vi "adaptive filter NLMS(sub VI).vi"(0 "ERR":dbl=0.060310676968585164, 1 "NLMS-r(防止過大步長)":dbl=10.0, 2 "輸入訊號":dbl, 3 "order":i32=10, 5 "u(收斂係數)":dbl=0.001) -> (6 "FIR輸出":dbl=-1.0516183080382016, 7 "收斂係數u":dbl=0.060310676968585164, 8 "權重":dbl[](array[numeric]))   [LabVIEW 2010]
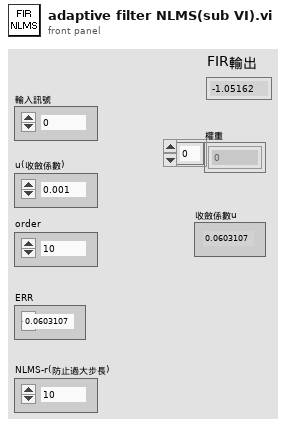
[diagram p1: front panel]
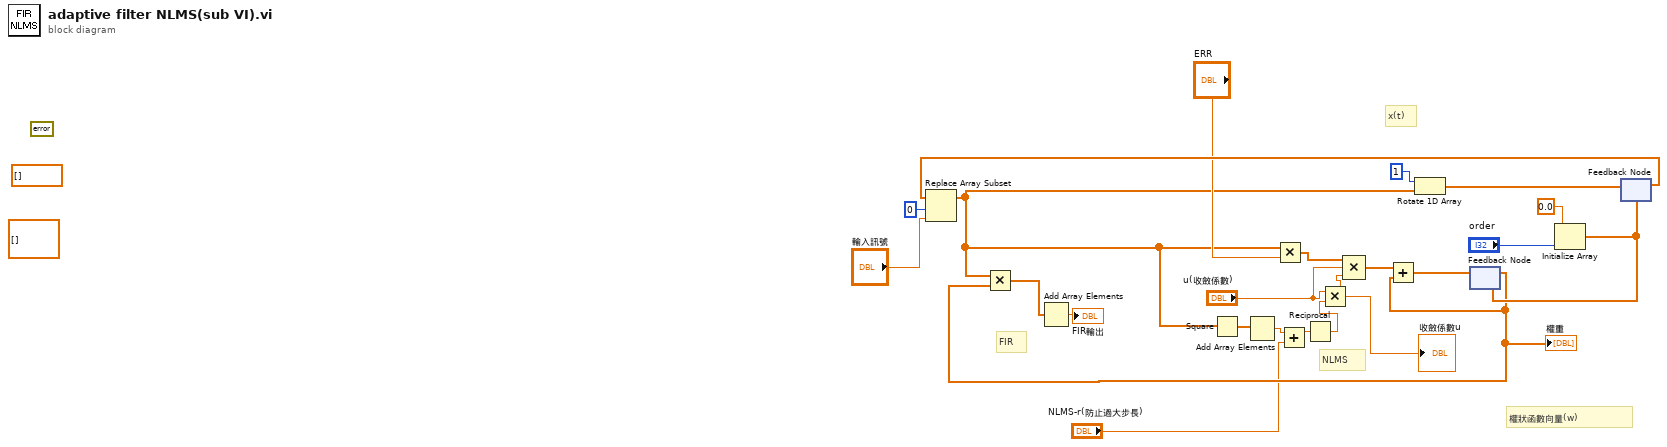
[diagram p0: block diagram]
diagram:
  (unwired) dbl[][] [] ("History Data")
  (unwired) dbl[] [] ("History Data")
  (unwired) errorcluster {"status"=FALSE, "code"=0, "source"=""} ("error constant")
  # "NLMS"
  # "FIR"
  # "權狀函數向量(w)"
  # "x(t)"
  n1 = Initialize Array(0.0 ("element"), "order") -> (w11:dbl[])
  n2 = feedback #1(w11) -> (w9:dbl[])
  "權重" <- w9
  n3 = feedback #2(w11) -> (w16:dbl[])
  n4 = Replace Array Subset(array=w16, new element="輸入訊號", index=0) -> (w8:dbl[])
  n5 = Multiply(x=w8, y=w9) -> (x*y=w19:dbl[])
  n6 = Add Array Elements(numeric array=w19) -> (sum=→"FIR輸出":dbl)
  n7 = Square(x=w8) -> (x^2=w7:dbl[])
  n8 = Add Array Elements(numeric array=w7) -> (sum=w6:dbl)
  n9 = Multiply(x=w8, y="ERR") -> (x*y=w23:dbl[])
  n10 = Add(x=w6, y="NLMS-r(防止過大步長)") -> (x+y=w4:dbl)
  n11 = Reciprocal(x=w4) -> (1/x=w2:dbl)
  n12 = Multiply(x="u(收斂係數)", y=w2) -> (x*y=w1:dbl)
  "收斂係數u" <- w1
  n13 = Compound Arithmetic op=MULTIPLY(w23, "u(收斂係數)", w1) -> (w12:dbl[])
  n14 = Add(x=w12, y=w9) -> (x+y=w13:dbl[])
  n15 = Rotate 1D Array(1:w8, 2:1 ("n")) -> (0:w17:dbl[])
  n16 = feedback-in #1(w13) -> ()
  n17 = feedback-in #2(w17) -> ()
